vi "ShrimpCam_Close.vi"(2 "Error In":errorcluster, 3 "Ref (cam in)":refnum<k24>) -> (0 "Error Out":errorcluster)   [LabVIEW 2018]
uses:
  C:/Users/user/Desktop/Thorcam/uc480DotNet.dll
  Thorcam/uc480DotNet.dll
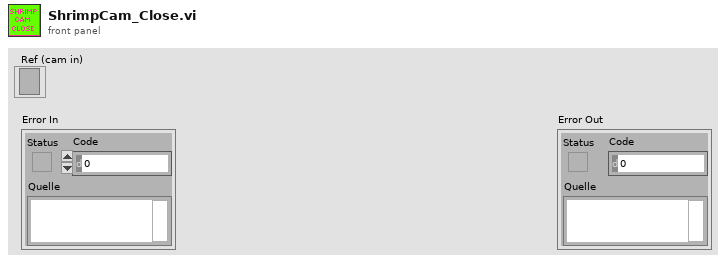
[diagram p1: front panel]
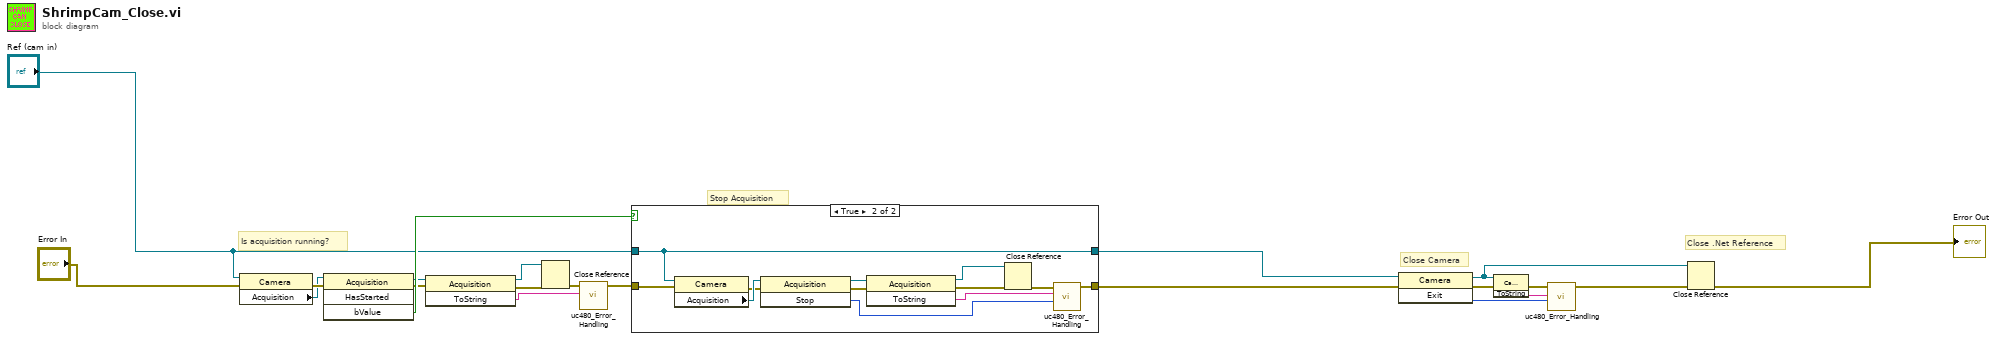
[diagram p0: block diagram]
diagram:
  # "Close .Net Reference"
  # "Is acquisition running?"
  # "Stop Acquisition"
  # "Close Camera"
  n1 = property class="Camera"(reference="Ref (cam in)", error in="Error In") -> (error out=w15:errorcluster, "Acquisition"=w14:refnum<k24>)  [unwired: 1 out]
  n2 = invoke class="Acquisition" method="HasStarted"(reference=w14, error in=w15) -> (reference out=w9:refnum<k24>, error out=w11:errorcluster, "bValue"=w13:bool)  [unwired: 2 in, 1 out]
  n3 = invoke class="Acquisition" method="ToString"(reference=w9, error in=w11) -> (reference out=w4:refnum<k24>, error out=w6:errorcluster, "ToString"=w10:string)  [unwired: 1 in]
  n4 = Close Reference(reference=w4, error in (no error)=w6) -> (error out=w5:errorcluster)
  n5 = call "uc480_Error_Handling.vi"("Error String"=w10, "Error In"=w5) -> ("Error Out"=w12:errorcluster)  [unwired: 9 in]
  n6 = case shown="True" w13 {
    tunnel: [w23 w34] -> w7
    tunnel: w12 -> [w23 w35]
    tunnel: "Ref (cam in)" -> [w22 w27]
    tunnel: [w22 w27] -> w8
    frame False {
    }
    frame True {
      n7 = property class="Camera"(reference=w27, error in=w35) -> (error out=w31:errorcluster, "Acquisition"=w32:refnum<k24>)  [unwired: 1 out]
      n8 = invoke class="Acquisition" method="Stop"(reference=w32, error in=w31) -> (reference out=w29:refnum<k24>, error out=w30:errorcluster, "Stop"=w28:i32)  [unwired: 1 in]
      n9 = invoke class="Acquisition" method="ToString"(reference=w29, error in=w30) -> (reference out=w24:refnum<k24>, error out=w26:errorcluster, "ToString"=w33:string)  [unwired: 1 in]
      n10 = Close Reference(reference=w24, error in (no error)=w26) -> (error out=w25:errorcluster)
      n11 = call "uc480_Error_Handling.vi"("Error Code"=w28, "Error String"=w33, "Error In"=w25) -> ("Error Out"=w34:errorcluster)  [unwired: 8 in]
    }
  }
  n12 = invoke class="Camera" method="Exit"(reference=w8, error in=w7) -> (reference out=w16:refnum<k24>, error out=w19:errorcluster, "Exit"=w18:i32)  [unwired: 1 in]
  n13 = invoke class="Camera" method="ToString"(reference=w16, error in=w19) -> (error out=w20:errorcluster, "ToString"=w21:string)  [unwired: 1 in, 1 out]
  n14 = call "uc480_Error_Handling.vi"("Error Code"=w18, "Error String"=w21, "Error In"=w20) -> ("Error Out"=w17:errorcluster)  [unwired: 8 in]
  n15 = Close Reference ("Close Referenz")(reference=w16, error in (no error)=w17) -> (error out=→"Error Out":errorcluster)
